vi "test Verify Hello LUnit.vi"(8 "error in":errorcluster, 11 "Test Case In":refnum<class "LUnit Extensions Tests.lvclass">) -> (0 "error out":errorcluster, 3 "Test Case Out":refnum<class "LUnit Extensions Tests.lvclass">)   [LabVIEW 2026, in "LUnit Extensions Tests.lvclass"]
uses:
  LUnit Extensions Tests.lvclass
  Source/Approval Tests/Options/Options.lvclass/Options.ctl
  Source/Approval Tests/Naming Data/Naming Data.lvclass/Naming Data.ctl
  <vilib>/Astemes/LUnit/Test Case.lvclass/Test Case.ctl
  240f995d-3744-484a-8956-6f48e6079b93.vi
  240f995d-3744-484a-8956-6f48e6079b93.vi/1e051690-6811-4db0-8b8f-f6ad9423d026.vi
  Source/Approval Tests/Replace if Empty.vi
  <vilib>/Astemes/LUnit/Palette/Pass If.vi
  Source/Approval Tests/Update Test Name if Not Defined.vi
  Source/Approval Tests/Verify Core.vi
  240f995d-3744-484a-8956-6f48e6079b93.vi/1e051690-6811-4db0-8b8f-f6ad9423d026.vi/93c5622b-9fb7-41e0-8c76-3fde37e94e34.vi
  Source/Approval Tests/Options/Read Scrubber.vi
  <vilib>/Astemes/LUnit/Core/LUnit Test Case/Private/Append Fail Result.vi
  <vilib>/Astemes/LUnit/Core/LUnit Test Case/Private/Append Pass Result.vi
  Source/Approval Tests/Naming Data/Read Test VI Name.vi
  Source/Approval Tests/Naming Data/Write Test VI Name.vi
  Source/Approval Tests/Options/Read Namer.vi
  Source/Approval Tests/Options/Read Naming Data.vi
  Source/Approval Tests/Options/Read Reporter.vi
  Source/Approval Tests/Options/Read Text Comparator.vi
  240f995d-3744-484a-8956-6f48e6079b93.vi/1e051690-6811-4db0-8b8f-f6ad9423d026.vi/93c5622b-9fb7-41e0-8c76-3fde37e94e34.vi/04cb982b-2eda-40d0-8d7e-90f8e0b569b2.vi
  <vilib>/Astemes/LUnit/Core/LUnit Test Case/Private/Run In UI.vi
  <vilib>/Utility/error.llb/Clear Errors.vi
  Source/Approval Tests/Options/Add Label to Namer.vi
  Source/Approval Tests/conv EOL.vi
  <vilib>/Utility/libraryn.llb/Check if File or Folder Exists.vi
  Source/Approval Tests/Reporter/Report.vi
  Source/Approval Tests/Options/Options.lvclass
  Source/Approval Tests/Scrubber/Scrubber.lvclass
  Source/Approval Tests/Namer/Namer.lvclass
  Source/Approval Tests/Naming Data/Naming Data.lvclass
  Source/Approval Tests/Reporter/Reporter.lvclass
  Source/Approval Tests/Text Comparator/Text Comparator.lvclass
  LUnit Extensions Tests.lvclass/LUnit Extensions Tests.ctl
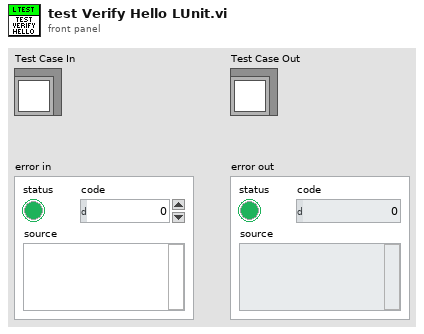
[diagram p1: front panel]
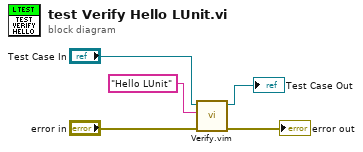
[diagram p0: block diagram]
diagram:
  n1 = call "Verify.vim"("error in"="error in", "Test Data"="Hello LUnit", "LUnit Test Case In"="Test Case In") -> ("error out"=→"error out":errorcluster, "LUnit Test Case Out"=→"Test Case Out":refnum<class "LUnit Extensions Tests.lvclass">)  [unwired: 7 in]
